vi "sv_Check for Continuous Swept Settings.vi"(0 "data to process":waveform(dbl)[](array[waveform]), 5 "channel index":i32, 11 "error in (no error)":errorcluster) -> (4 "data to process out":waveform(dbl)[](array[waveform]), 6 "chirp settings":T1={"amplitude"=0.0, "frequency range"={"start (Hz)"=20.0, "stop (Hz)"=20000.0, "frequency spacing"=enum."Logarithmic"}, "sampling info"={"Fs"=50000.0, "chirp duration [s]"=3.0}, "initial states"={"frequency [Hz]"=20.0, "phase [rad]"=0.0, "elapsed time [s]"=0.0}, "frequency slope"=0.0, "maximum harmonic"=0, "prefix len [samples]"={"integer"=0, "fractional"=0.0}} {"frequency slope" format="%.2f"; "prefix len [samples]"."fractional" format="%.2p"; "initial states"."elapsed time [s]" format="%.2f"; "initial states"."phase [rad]" format="%.2f"; "initial states"."frequency [Hz]" format="%.2f"; "sampling info"."chirp duration [s]" format="%.2f"; "sampling info"."Fs" format="%.2p"; "frequency range"."stop (Hz)" format="%.2f"; "frequency range"."start (Hz)" format="%.2f"; "amplitude" format="%.2f"}, 15 "error out":errorcluster)   [LabVIEW 2017, in "SoundVib_ContSweptSine.lvlib"]
uses:
  <vilib>/addons/Sound and Vibration/svt_Continuous Swept Sine/SoundVib_ContSweptSine.lvlib
  <vilib>/addons/_NISVFA/_Generation/subVIs/sv_Chirp Settings.ctl
  <vilib>/addons/_NISVFA/_Generation/SoundVib_Generation.lvlib
panel:
  in  "chirp settings":T1={"amplitude"=0.0, "frequency range"={"start (Hz)"=20.0, "stop (Hz)"=20000.0, "frequency spacing"=enum."Logarithmic"}, "sampling info"={"Fs"=50000.0, "chirp duration [s]"=3.0}, "initial states"={"frequency [Hz]"=20.0, "phase [rad]"=0.0, "elapsed time [s]"=0.0}, "frequency slope"=0.0, "maximum harmonic"=0, "prefix len [samples]"={"integer"=0, "fractional"=0.0}} {"frequency slope" format="%.2f"; "prefix len [samples]"."fractional" format="%.2p"; "initial states"."elapsed time [s]" format="%.2f"; "initial states"."phase [rad]" format="%.2f"; "initial states"."frequency [Hz]" format="%.2f"; "sampling info"."chirp duration [s]" format="%.2f"; "sampling info"."Fs" format="%.2p"; "frequency range"."stop (Hz)" format="%.2f"; "frequency range"."start (Hz)" format="%.2f"; "amplitude" format="%.2f"}
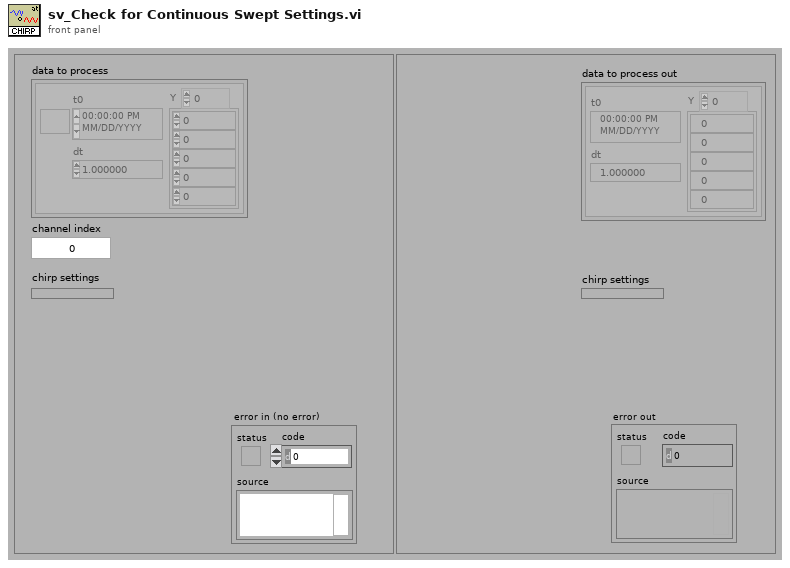
[diagram p1: front panel]
types:
  T1 = typedef "SoundVib_Generation.lvlib/sv_Chirp Settings.ctl" = cluster{"amplitude":dbl, "frequency range":cluster{"start (Hz)":dbl, "stop (Hz)":dbl, "frequency spacing":enum16{"Linear", "Logarithmic"}}, "sampling info":cluster{"Fs":dbl, "chirp duration [s]":dbl}, "initial states":cluster{"frequency [Hz]":dbl, "phase [rad]":dbl, "elapsed time [s]":dbl}, "frequency slope":dbl, "maximum harmonic":i32, "prefix len [samples]":cluster{"integer":u32, "fractional":dbl}}
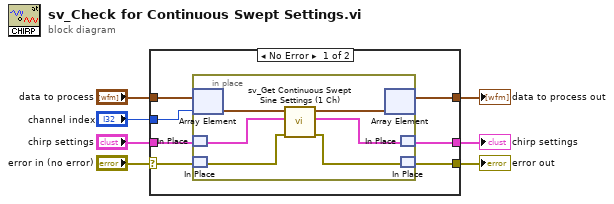
[diagram p0: block diagram]
diagram:
  n1 = case shown="No Error" "error in (no error)" {
    selector: "error in (no error)" -> [w12 w23]
    tunnel: [w11 w23] -> w6
    tunnel: "chirp settings" -> [w14 w22]
    tunnel: "data to process" -> [w10 w21]
    tunnel: [w9 w21] -> w3
    tunnel: [w13 w22] -> w2
    tunnel: "channel index" -> [w8 _]
    frame No Error {
      n2 = in-place {
        n3 = in-place-array #1(w10, w8) -> (w20:waveform(dbl))
        n4 = in-place-match #2(w14) -> (w18:T1)
        n5 = in-place-match #3(w12) -> (w15:errorcluster)
        n6 = call <vilib>:"sv_Get Continuous Swept Sine Settings (1 Ch).vi"("error in (no error)"=w15, "chirp settings in"=w18, "waveform"=w20) -> ("error out"=w16:errorcluster, "chirp settings out"=w17:T1, "same waveform"=w19:waveform(dbl))  [unwired: 6 in]
        n7 = in-place-array #1(w19) -> (w9:waveform(dbl)[])  [unwired: 1 out]
        n8 = in-place-match #2(w17) -> (w13:T1)
        n9 = in-place-match #3(w16) -> (w11:errorcluster)
      }
    }
    frame Error {
    }
  }
  "error out" <- w6
  "data to process out" <- w3
  "chirp settings" <- w2
